vi "去除无效数据_整数.vi"(0 "关联成像原理":i32[](array[numeric]), 5 "光源散斑类型":i32[](array[numeric]), 7 "图像类型":i32[](array[numeric]), 9 "重建方法":i32[](array[numeric]), 11 "优化算法":i32[](array[numeric])) -> (4 "关联成像原理最终选择":i32, 6 "光源散斑类型最终选择":i32, 8 "图像类型最终选择":i32, 10 "重建方法最终选择":i32, 15 "优化算法最终选择":i32)   [LabVIEW 2018]
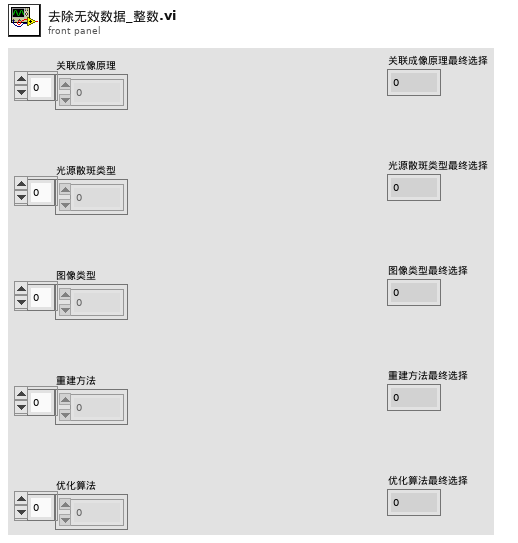
[diagram p1: front panel]
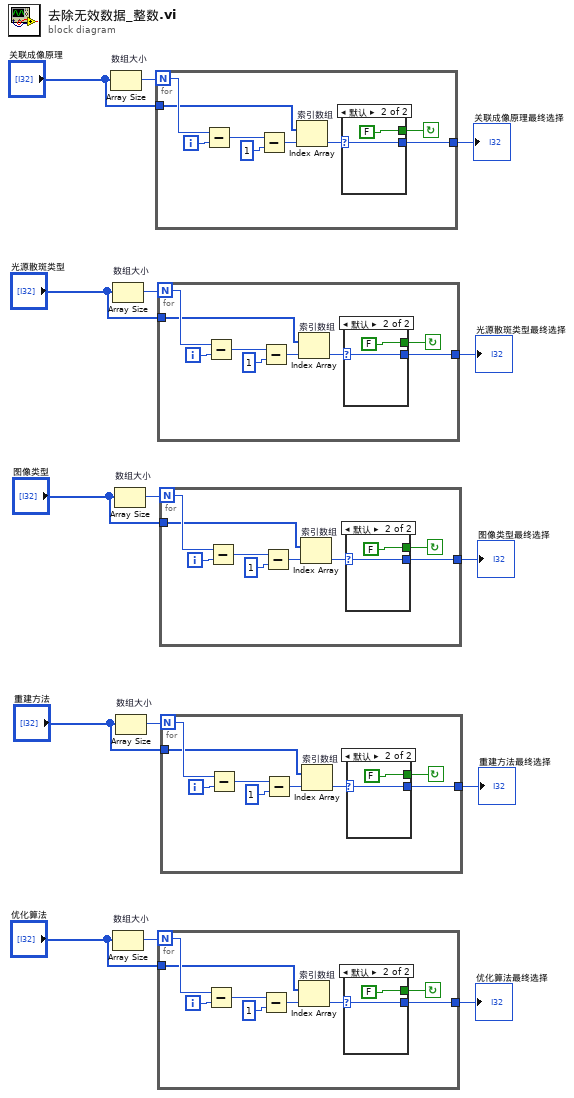
[diagram p0: block diagram]
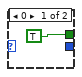
[diagram p2: hidden frame]
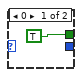
[diagram p3: hidden frame]
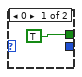
[diagram p4: hidden frame]
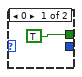
[diagram p5: hidden frame]
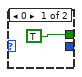
[diagram p6: hidden frame]
diagram:
  n1 = Array Size "数组大小"(array="关联成像原理") -> (size(s)=w15:i32)
  n2 = Array Size "数组大小"(array="光源散斑类型") -> (size(s)=w12:i32)
  n3 = Array Size "数组大小"(array="优化算法") -> (size(s)=w3:i32)
  n4 = Array Size "数组大小"(array="图像类型") -> (size(s)=w9:i32)
  n5 = Array Size "数组大小"(array="重建方法") -> (size(s)=w6:i32)
  n6 = for {
    N: w15 -> [w24]
    tunnel: [w17] -> w13
    tunnel: "关联成像原理" -> [w16]
    i -> [w23]
    stop <- w18 continue-if-true
    n7 = Subtract(x=w24, y=w23) -> (x-y=w22:i32)
    n8 = Subtract(x=w22, y=1) -> (x-y=w20:i32)
    n9 = Index Array "索引数组"(array=w16, index=w20) -> (element=w19:i32)
    n10 = case shown="默认" w19 {
      selector: w19 -> [_ w26]
      tunnel: [TRUE FALSE] -> w18
      tunnel: [_ w26] -> w17
      frame 0 {
      }
      frame Default {
      }
    }
  }
  "关联成像原理最终选择" <- w13
  n11 = for {
    N: w12 -> [w36]
    tunnel: [w29] -> w10
    tunnel: "光源散斑类型" -> [w28]
    i -> [w35]
    stop <- w30 continue-if-true
    n12 = Subtract(x=w36, y=w35) -> (x-y=w34:i32)
    n13 = Subtract(x=w34, y=1) -> (x-y=w32:i32)
    n14 = Index Array "索引数组"(array=w28, index=w32) -> (element=w31:i32)
    n15 = case shown="默认" w31 {
      selector: w31 -> [_ w38]
      tunnel: [TRUE FALSE] -> w30
      tunnel: [_ w38] -> w29
      frame 0 {
      }
      frame Default {
      }
    }
  }
  "光源散斑类型最终选择" <- w10
  n16 = for {
    N: w3 -> [w48]
    tunnel: [w41] -> w1
    tunnel: "优化算法" -> [w40]
    i -> [w47]
    stop <- w42 continue-if-true
    n17 = Subtract(x=w48, y=w47) -> (x-y=w46:i32)
    n18 = Subtract(x=w46, y=1) -> (x-y=w44:i32)
    n19 = Index Array "索引数组"(array=w40, index=w44) -> (element=w43:i32)
    n20 = case shown="默认" w43 {
      selector: w43 -> [_ w50]
      tunnel: [TRUE FALSE] -> w42
      tunnel: [_ w50] -> w41
      frame 0 {
      }
      frame Default {
      }
    }
  }
  "优化算法最终选择" <- w1
  n21 = for {
    N: w9 -> [w60]
    tunnel: [w53] -> w7
    tunnel: "图像类型" -> [w52]
    i -> [w59]
    stop <- w54 continue-if-true
    n22 = Subtract(x=w60, y=w59) -> (x-y=w58:i32)
    n23 = Subtract(x=w58, y=1) -> (x-y=w56:i32)
    n24 = Index Array "索引数组"(array=w52, index=w56) -> (element=w55:i32)
    n25 = case shown="默认" w55 {
      selector: w55 -> [_ w62]
      tunnel: [TRUE FALSE] -> w54
      tunnel: [_ w62] -> w53
      frame 0 {
      }
      frame Default {
      }
    }
  }
  "图像类型最终选择" <- w7
  n26 = for {
    N: w6 -> [w72]
    tunnel: [w65] -> w4
    tunnel: "重建方法" -> [w64]
    i -> [w71]
    stop <- w66 continue-if-true
    n27 = Subtract(x=w72, y=w71) -> (x-y=w70:i32)
    n28 = Subtract(x=w70, y=1) -> (x-y=w68:i32)
    n29 = Index Array "索引数组"(array=w64, index=w68) -> (element=w67:i32)
    n30 = case shown="默认" w67 {
      selector: w67 -> [_ w74]
      tunnel: [TRUE FALSE] -> w66
      tunnel: [_ w74] -> w65
      frame 0 {
      }
      frame Default {
      }
    }
  }
  "重建方法最终选择" <- w4
